vi "PSCP.vi"(8 "error in":errorcluster, 10 "Host":string="172.22.11.2", 11 "pscp path":path=path "bin/pscp.exe") -> (0 "error out":errorcluster, 1 "return code":i32, 2 "Errors":string, 3 "Command Return Value(s)":string, 5 "Command Executed":string)   [LabVIEW 2016]
panel:
  in  "remote path":path=path "~/"
  in  "Files":path[](array[path])
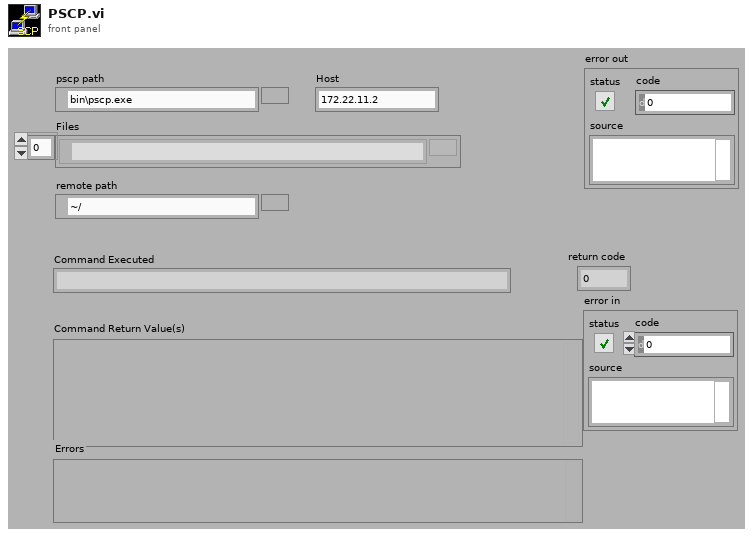
[diagram p1: front panel]
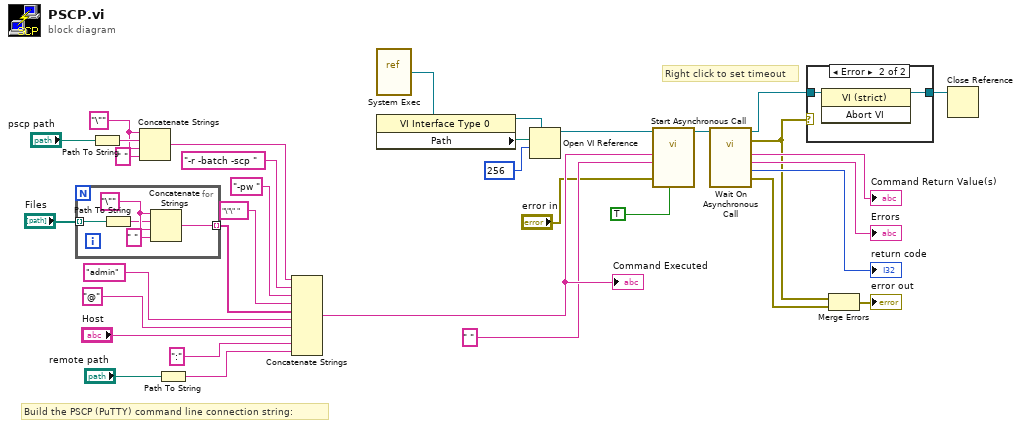
[diagram p0: block diagram]
diagram:
  w29 = "\"" ("string")
  # "Right click to set timeout"
  # "Build the PSCP (PuTTY) command line connection string:"
  n1 = for {
    tunnel: "Files" -> [w37] mode=indexing
    tunnel: [w35] -> w27 mode=indexing
    w39 = "\"" ("string")
    n2 = Path To String(path=w37) -> (string=w38:string)
    n3 = Concatenate Strings(w39, w38, w39, " " ("string")) -> (w35:string)
  }
  n4 = Path To String(path="pscp path") -> (string=w30:string)
  n5 = Concatenate Strings(w29, w30, w29, " " ("string")) -> (w26:string)
  n6 = Path To String(path="remote path") -> (string=w23:string)
  n7 = Concatenate Strings(w26, "-r -batch -scp " ("string"), "-pw " ("string"), "\"\" " ("Password"), w27, "admin" ("Username"), "@" ("string"), "Host", ":" ("string"), w23) -> (w12:string)
  "Command Executed" <- w12
  n8 = vi-ref <vilib>:"System Exec.vi"() -> (w17:refnum<vi>)
  n9 = property class="VI Interface Type 0"(reference=w17) -> (reference out=w14:refnum<vi>, "Path"=w16:path)  [unwired: 1 in, 1 out]
  n10 = Open VI Reference(type specifier VI Refnum (for type only)=w14, vi path=w16, options=256) -> (vi reference=w18:refnum<vi>)  [unwired: 3 in, 1 out]
  n11 = call-by-ref "Start Asynchronous Call"(reference=w18, "run minimized? (F)"=TRUE ("Hide DOS\nWindow?"), "error in (no error)"="error in", "standard input"=" ", "command line"=w12) -> (reference out=w13:refnum<vi>)  [unwired: 5 in, 5 out]
  n12 = call-by-ref "Wait On Asynchronous Call"(reference=w13) -> (reference out=w2:refnum<vi>, error out=w1:errorcluster, 0:"error out"=w4:errorcluster, "return code"=→"return code":i32, "standard error"=→"Errors":string, "standard output"=→"Command Return Value(s)":string)  [unwired: 9 in]
  n13 = case shown="Error" w1 {
    tunnel: [w40 w42] -> w3
    tunnel: w2 -> [w40 w41]
    frame No Error {
    }
    frame Error {
      n14 = invoke class="VI (strict)" method="Abort VI"(reference=w41) -> (reference out=w42:refnum<vi>)  [unwired: 2 in, 2 out]
    }
  }
  n15 = Merge Errors(w1, w4) -> (→"error out":errorcluster)
  n16 = Close Reference(reference=w3) -> ()  [unwired: 1 in, 1 out]
